vi "Show_Test_Currents.vi"() -> ()   [LabVIEW 2016]
uses:
  Hall Effect Library/Hall Effect Library.lvlib
panel:
  out "6-Contact Sample Hall Measurements":T1 {"I8" format="%#_6e"; "I7" format="%#_6e"; "I6" format="%#_6e"; "I5" format="%#_6e"; "I4" format="%#_6e"; "I3" format="%#_6e"; "I2" format="%#_6e"; "I1" format="%#_6e"}
  out "Hall Measurements":T1 {"I8" format="%#_6e"; "I7" format="%#_6e"; "I6" format="%#_6e"; "I5" format="%#_6e"; "I4" format="%#_6e"; "I3" format="%#_6e"; "I2" format="%#_6e"; "I1" format="%#_6e"}
  in  "OK Button":bool
  out "8-Contact Sample Hall Measurements":cluster{"I1":dbl, "I2":dbl, "I3":dbl, "I4":dbl} {"I4" format="%#_6e"; "I3" format="%#_6e"; "I2" format="%#_6e"; "I1" format="%#_6e"}
  out "8-Contact Sample Resistivity Measurements":cluster{"I1":dbl, "I2":dbl, "I3":dbl, "I4":dbl} {"I4" format="%#_6e"; "I3" format="%#_6e"; "I2" format="%#_6e"; "I1" format="%#_6e"}
  out "6-Contact Sample Resistivity Measurements":cluster{"I1":dbl, "I2":dbl, "I3":dbl, "I4":dbl} {"I4" format="%#_6e"; "I3" format="%#_6e"; "I2" format="%#_6e"; "I1" format="%#_6e"}
  out "Bar Sample Hall Measurements":cluster{"Bar Sample Hall Current":dbl} {"Bar Sample Hall Current" format="%#_6e"}
  out "Bar Sample Resistivity Measurements":cluster{"Bar Sample Resistivity Current":dbl} {"Bar Sample Resistivity Current" format="%#_6e"}
  out "Van Der Pauw Measurements":T1 {"I8" format="%#_6e"; "I7" format="%#_6e"; "I6" format="%#_6e"; "I5" format="%#_6e"; "I4" format="%#_6e"; "I3" format="%#_6e"; "I2" format="%#_6e"; "I1" format="%#_6e"}
  # "Current"
  # "Pos"
  # "Amps"
  # "Neg"
  # "Direction"
  # "Amps"
  # "Current"
  # "Pos"
  # "Amps"
  # "Neg"
  # "Direction"
  # "Current"
  # "Pos"
  # "Amps"
  # "Neg"
  # "Direction"
  # "Current"
  # "Pos"
  # "Amps"
  # "Neg"
  # "Direction"
  # "Ih"
  # "Amps"
  # "Ir"
  # "Amps"
  # "Amps"
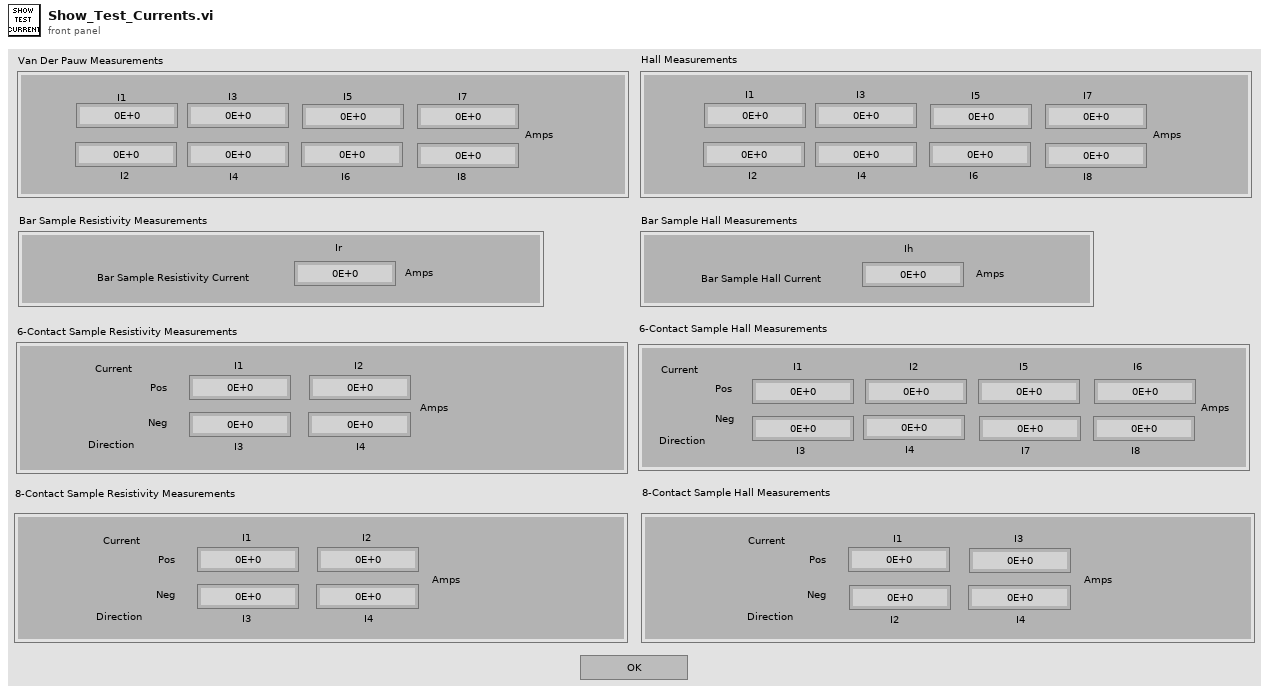
[diagram p1: front panel]
types:
  T1 = cluster{"I1":dbl, "I2":dbl, "I3":dbl, "I4":dbl, "I5":dbl, "I6":dbl, "I7":dbl, "I8":dbl}
  T2 = cluster{"Bar Sample Resistivity Currents[0]":dbl}
  T3 = cluster{"Hall Effect Currents[0]":dbl, "Hall Effect Currents[1]":dbl, "Hall Effect Currents[2]":dbl, "Hall Effect Currents[3]":dbl, "Hall Effect Currents[4]":dbl, "Hall Effect Currents[5]":dbl, "Hall Effect Currents[6]":dbl, "Hall Effect Currents[7]":dbl}
  T4 = cluster{"Van Der Pauw Currents[0]":dbl, "Van Der Pauw Currents[1]":dbl, "Van Der Pauw Currents[2]":dbl, "Van Der Pauw Currents[3]":dbl, "Van Der Pauw Currents[4]":dbl, "Van Der Pauw Currents[5]":dbl, "Van Der Pauw Currents[6]":dbl, "Van Der Pauw Currents[7]":dbl}
  T5 = cluster{"8-Contact Sample Resistivity Currents[0]":dbl, "8-Contact Sample Resistivity Currents[1]":dbl, "8-Contact Sample Resistivity Currents[2]":dbl, "8-Contact Sample Resistivity Currents[3]":dbl}
  T6 = cluster{"6-Contact Sample Resistivity Currents[0]":dbl, "6-Contact Sample Resistivity Currents[1]":dbl, "6-Contact Sample Resistivity Currents[2]":dbl, "6-Contact Sample Resistivity Currents[3]":dbl}
  T7 = cluster{"8-Contact Sample Hall Currents[0]":dbl, "8-Contact Sample Hall Currents[1]":dbl, "8-Contact Sample Hall Currents[2]":dbl, "8-Contact Sample Hall Currents[3]":dbl}
  T8 = cluster{"6-Contact Sample Hall Currents[0]":dbl, "6-Contact Sample Hall Currents[1]":dbl, "6-Contact Sample Hall Currents[2]":dbl, "6-Contact Sample Hall Currents[3]":dbl, "6-Contact Sample Hall Currents[4]":dbl, "6-Contact Sample Hall Currents[5]":dbl, "6-Contact Sample Hall Currents[6]":dbl, "6-Contact Sample Hall Currents[7]":dbl}
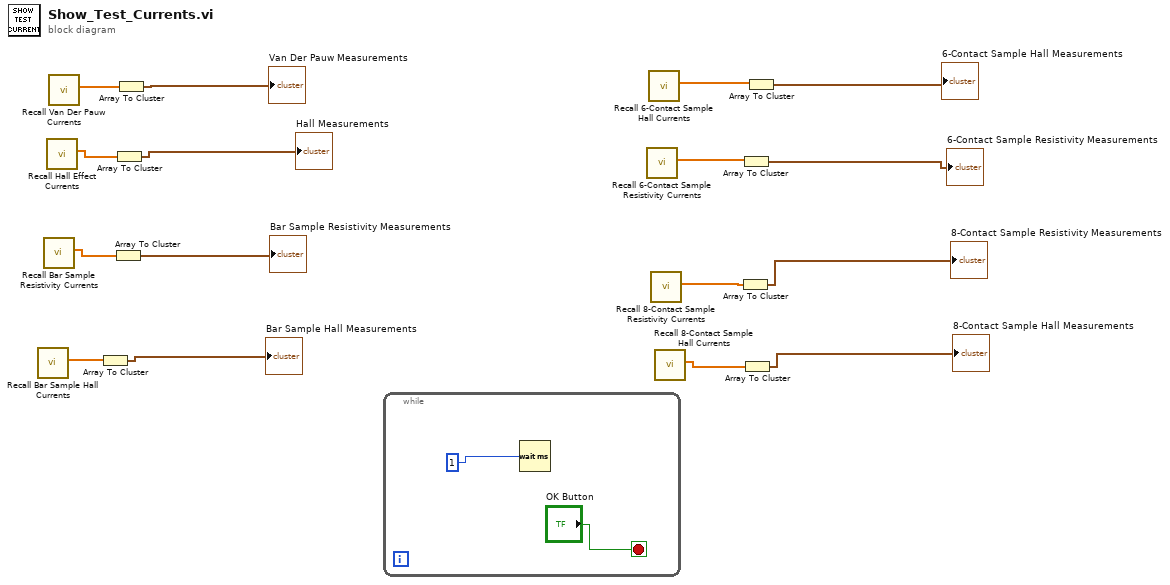
[diagram p0: block diagram]
diagram:
  n1 = call "Recall Bar Sample Hall Currents.vi"() -> ("Bar Sample Hall Currents"=w11:dbl[])  [unwired: 11 in]
  n2 = call "Recall Bar Sample Resistivity Currents.vi"() -> ("Bar Sample Resistivity Currents"=w13:dbl[])  [unwired: 11 in]
  n3 = call "Recall Hall Effect Currents.vi"() -> ("Hall Effect Currents"=w14:dbl[])  [unwired: 11 in]
  n4 = call "Recall Van Der Pauw Currents.vi"() -> ("Van Der Pauw Currents"=w16:dbl[])  [unwired: 11 in]
  n5 = Array To Cluster(array=w11) -> (cluster=→"Bar Sample Hall Measurements":cluster{"Bar Sample Hall Currents[0]":dbl})
  n6 = Array To Cluster(array=w13) -> (cluster=→"Bar Sample Resistivity Measurements":T2)
  n7 = Array To Cluster(array=w14) -> (cluster=→"Hall Measurements":T3)
  n8 = Array To Cluster(array=w16) -> (cluster=→"Van Der Pauw Measurements":T4)
  n9 = while {
    stop <- "OK Button" stop-if-true
    n10 = Wait (ms)(milliseconds to wait=1) -> ()  [unwired: 1 out]
  }
  n11 = call "Recall 6-Contact Sample Resistivity Currents.vi"() -> ("6-Contact Sample Resistivity Currents"=w8:dbl[])  [unwired: 11 in]
  n12 = call "Recall 6-Contact Sample Hall Currents.vi"() -> ("6-Contact Sample Hall Currents"=w9:dbl[])  [unwired: 11 in]
  n13 = call "Recall 8-Contact Sample Resistivity Currents.vi"() -> ("8-Contact Sample Resistivity Currents"=w6:dbl[])  [unwired: 11 in]
  n14 = call "Recall 8-Contact Sample Hall Currents.vi"() -> ("8-Contact Sample Hall Currents"=w4:dbl[])  [unwired: 11 in]
  n15 = Array To Cluster(array=w6) -> (cluster=→"8-Contact Sample Resistivity Measurements":T5)
  n16 = Array To Cluster(array=w8) -> (cluster=→"6-Contact Sample Resistivity Measurements":T6)
  n17 = Array To Cluster(array=w4) -> (cluster=→"8-Contact Sample Hall Measurements":T7)
  n18 = Array To Cluster(array=w9) -> (cluster=→"6-Contact Sample Hall Measurements":T8)
